vi "get data definition.vi"(10 "channel classification":T1, 11 "fixed channel runtime in":refnum<class "control module runtime.lvclass">) -> (1 "valid?":bool, 2 "index cluster":variant, 3 "fixed channel runtime out":refnum<class "control module runtime.lvclass">)   [LabVIEW 2013, in "control module runtime.lvclass"]
uses:
  control module runtime.lvclass
  <vilib>/NI/Tag Bus Module Framework/channel/channel classification.ctl
  <vilib>/NI/Tag Bus Module Framework/channel/TBM channel.lvclass
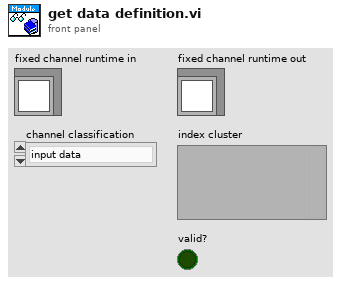
[diagram p1: front panel]
types:
  T1 = typedef "TBM channel.lvclass/channel classification.ctl" = enum16{"input data", "output data", "processing parameter", "processing result"}
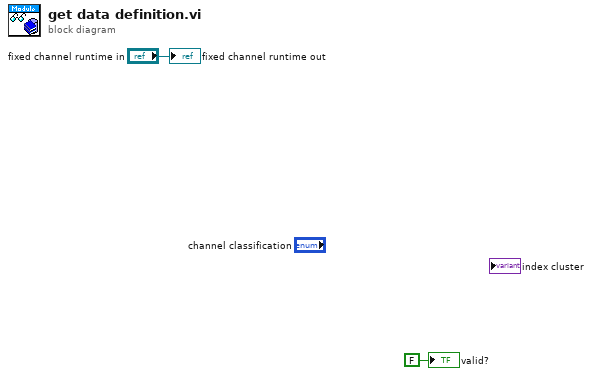
[diagram p0: block diagram]
diagram:
  "fixed channel runtime out" <- "fixed channel runtime in"
  "valid?" <- FALSE ("valid?")
